vi "LS372_Ch2.vi"   [LabVIEW 2018]
uses:
  Instrument_Setup.vi
  Equipment/Lake Shore 372/Lake Shore 372.lvlib
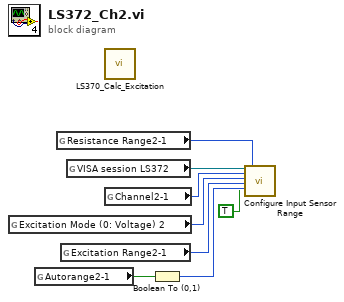
[diagram p0: block diagram]
diagram:
  n1 = global read "Instrument_Setup.vi" "Excitation Mode (0: Voltage) 2"() -> (w4:u16)
  n2 = global read "Instrument_Setup.vi" "Autorange2-1"() -> (w8:bool)
  n3 = global read "Instrument_Setup.vi" "Resistance Range2-1"() -> (w2:u16)
  n4 = global read "Instrument_Setup.vi" "Excitation Range2-1"() -> (w3:u16)
  n5 = global read "Instrument_Setup.vi" "VISA session LS372"() -> (w1:refnum<visa-resource-name>)
  n6 = call "LS370_Calc_Excitation.vi"() -> ()  [unwired: 12 in]
  n7 = global read "Instrument_Setup.vi" "Channel2-1"() -> (w6:u16)
  n8 = Boolean To (0,1)(Boolean=w8) -> (0, 1=w7:i16)
  n9 = call "Configure Input Sensor Range.vi"("VISA resource name"=w1, "Channel (1)"=w6, "Excitation Mode (0: Voltage)"=w4, "Excitation Range (5: 200 uV / 100 pA)"=w3, "Autorange (0: Autorange off)"=w7, "Resistance Range (17: 200 kOhm)"=w2, "Excitation  (T: On)"=TRUE) -> ()  [unwired: 11 in, 2 out]
